vi "WriteU32.vi"(10 "Data":u32, 11 "Address":u32) -> ()   [LabVIEW 2016]
uses:
  <vilib>/rvi/Memory/Memory_Emulation/nirvimemoryFastEmulation.vi
  <vilib>/rvi/Memory/Memory_Emulation/nirvimemoryEmulation.vi
  <vilib>/rvi/Emulation/niFpgaEmulationIsFPGAContextNoSignature.vi
  <vilib>/rvi/DataTransferAndStorage/Container/Common/niFpgaContainerGetUniqueNameForEmu.vi
  <vilib>/rvi/Emulation/niFpgaProcessEmulError.vi
  <vilib>/rvi/Emulation/niFpgaSctlEmulationGetInTimedLoop.vi
  <vilib>/rvi/errors/nirviReportUnexpectedCaseInternalError (U32).vi
  <vilib>/rvi/DataTransferAndStorage/Container/Common/niFpgaContainerExecOnDevCompGetState.vi
  <vilib>/rvi/Memory/Memory_Emulation/niFpgaMemoryEmulationCacheClearOnFirstRun.vi
  <vilib>/rvi/Memory/Memory_Emulation/nirvimemoryEmulationManagerCache_MakeExclusive.vi
  <vilib>/rvi/Memory/Memory_Emulation/niFpgaMemoryEmulationValidateCache.vi
  <vilib>/rvi/Memory/Memory_Emulation/nirvimemoryEmulationManagerCache_InsertValue.vi
  <vilib>/Utility/error.llb/Clear Errors.vi
  <vilib>/rvi/Memory/Memory_Emulation/nirvimemoryEmulationManagerCache_ReleaseExclusive.vi
  <vilib>/rvi/Memory/Memory_Emulation/nirvimemoryEmulationManagerCache_GetValue.vi
  <vilib>/rvi/Memory/Memory_Emulation/nirvimemoryEmulationManagerCache_SetValue.vi
  <vilib>/rvi/Emulation/niFpgaSctlEmulationResourceMgr.vi
  <vilib>/rvi/DataTransferAndStorage/Container/XNode/niFpgaContainer.xnode
  <vilib>/rvi/Memory/Memory_Emulation/niFpgaMemoryEmulationRefIn.vi
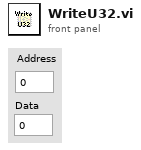
[diagram p1: front panel]
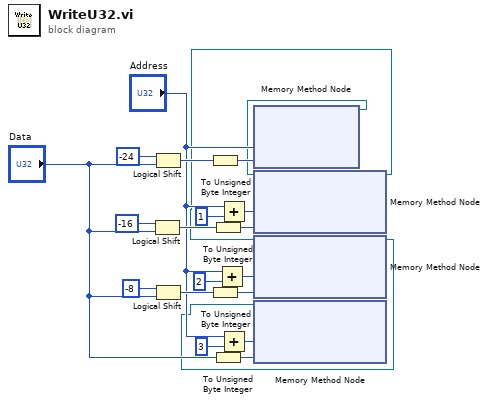
[diagram p0: block diagram]
diagram:
  n1 = Logical Shift(y=i16 -16, x="Data") -> (x << y=w6:u32)
  n2 = Logical Shift(y=i16 -24, x="Data") -> (x << y=w17:u32)
  n3 = Logical Shift(y=i16 -8, x="Data") -> (x << y=w14:u32)
  n4 = To Unsigned Byte Integer(number=w17) -> (unsigned 8bit integer=w18:u8)
  n5 = To Unsigned Byte Integer(number=w14) -> (unsigned 8bit integer=w13:u8)
  n6 = To Unsigned Byte Integer(number=w6) -> (unsigned 8bit integer=w16:u8)
  n7 = To Unsigned Byte Integer(number="Data") -> (unsigned 8bit integer=w15:u8)
  n8 = Add(x="Address", y=u32 2) -> (x+y=w8:u32)
  n9 = Add(x="Address", y=u32 1) -> (x+y=w21:u32)
  n10 = Add(x="Address", y=u32 3) -> (x+y=w10:u32)
  n11 = xnode ("Memory Method Node")("Address"="Address", "Data"=w18) -> ("Memory Out"=w3:refnum<k21>)  [unwired: 1 in]
  n12 = xnode ("Memory Method Node")("Address"=w21, "Data"=w16, "Memory In"=w3) -> ("Memory Out"=w2:refnum<k21>)
  n13 = xnode ("Memory Method Node")("Address"=w8, "Data"=w13, "Memory In"=w2) -> ("Memory Out"=w1:refnum<k21>)
  n14 = xnode ("Memory Method Node")("Address"=w10, "Data"=w15, "Memory In"=w1) -> ()  [unwired: 1 out]
